vi "sqr wave.vi"() -> ()   [LabVIEW 2020]
uses:
  <vilib>/express/express analysis/Spectral/Block/exnSpectralBlock spectral measurements RMS poly.vi
  <vilib>/express/express analysis/Spectral/Block/exnSpectralBlock spectral measurements RMS WFM.vi
  <vilib>/express/express analysis/Spectral/XNode/ExpressSpectralMeasurementsBlockNode.xnode
  <vilib>/measure/NI_MABase.lvlib
panel:
  in  "signal type":T1(ring)
  out "fft 2":cluster{"f0":dbl, "df":dbl, "magnitude":dbl[]}(graph)
  out "time analysis":waveform(dbl)(graph)
  out "k":dbl
  out "observation window":dbl
  out "frequency resolution":dbl
  in  "N":dbl
  in  "fs":dbl
  in  "frequency":dbl=10.0 format="%0.2p"
  in  "amplitude":dbl=1.0 format="%0.2p"
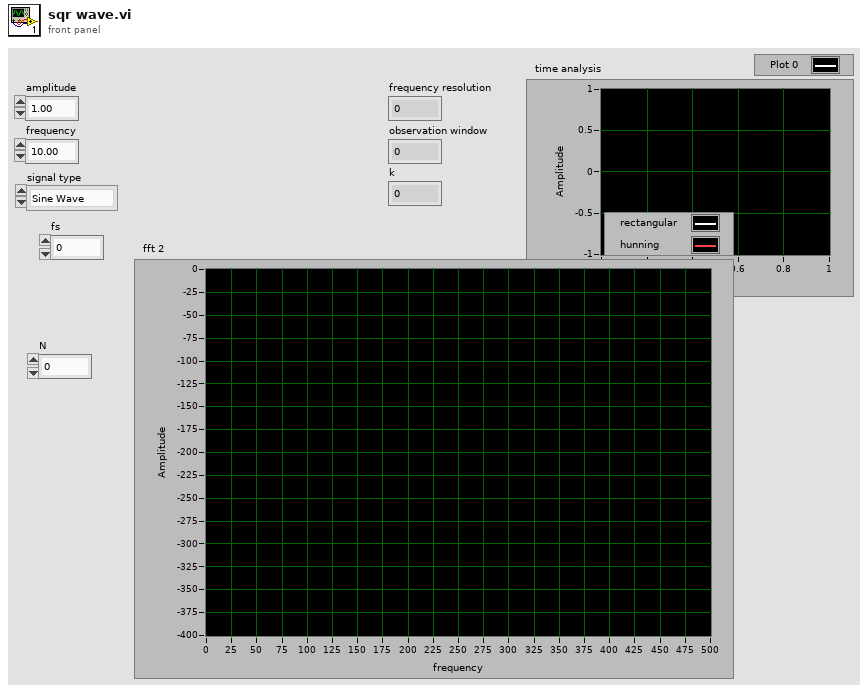
[diagram p1: front panel]
types:
  T1 = enum16{"Sine Wave", "Triangle Wave", "Square Wave", "Sawtooth Wave"}
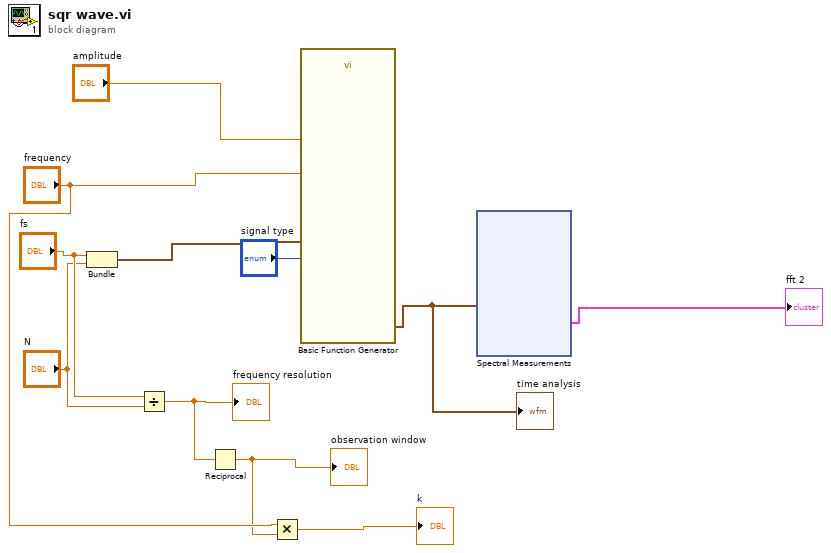
[diagram p0: block diagram]
diagram:
  n1 = Bundle("fs"="fs", "N"="N") -> (w10:cluster{"fs":dbl, "N":dbl})  [unwired: 1 in]
  n2 = Divide(x="fs", y="N") -> (x/y=w7:dbl)
  "frequency resolution" <- w7
  n3 = Reciprocal(x=w7) -> (1/x=w5:dbl)
  "observation window" <- w5
  n4 = Multiply(x="frequency", y=w5) -> (x*y=→"k":dbl)
  n5 = call <vilib>:"Basic Function Generator.vi"("sampling info"=w10, "signal type"="signal type", "amplitude"="amplitude", "frequency"="frequency") -> ("signal out"=w3:waveform(dbl))  [unwired: 5 in, 2 out]
  "time analysis" <- w3
  n6 = xnode "Spectral Measurements"("Signals"=w3) -> ("FFT - (RMS)"=→"fft 2":cluster{"f0":dbl, "df":dbl, "magnitude":dbl[]})  [unwired: 1 in, 2 out]
